vi "format_configuration_commands.vi"(8 "error in (no error)":errorcluster, 9 "True/false to 0/1?":bool, 10 "Configuration editables":T1(array[cluster])=[{"INI key name"="FieldCurrentRatio", "Configuration command"="CONF:COIL"}, {"INI key name"="HasPSwitch", "Configuration command"="CONF:PS"}, {"INI key name"="SwitchHtrCurrent", "Configuration command"="CONF:PS:CURR"}, {"INI key name"="SwitchWaitTime", "Configuration command"="CONF:PS:HTIME"}, {"INI key name"="SwitchWaitTime", "Configuration command"="CONF:PS:CTIME"}, {"INI key name"="SwitchCoolingGain", "Configuration command"="CONF:PS:CGAIN"}, {"INI key name"="StabilitySetting", "Configuration command"="CONF:STAB"}, {"INI key name"="MaxCurrent", "Configuration command"="CONF:CURR:RATING"}, {"INI key name"="MaxCurrent", "Configuration command"="CONF:CURR:LIM"}, {"INI key name"="LimitCurrent", "Configuration command"="CONF:CURR:LIM"}, {"INI key name"="QuenchDetectEnable", "Configuration command"="CONF:QU:DET"}, {"INI key name"="QuenchDetectRate", "Configuration command"="CONF:QU:RATE"}, {"INI key name"="AbsorberPresent", "Configuration command"="CONF:AB"}, {"INI key name"="SwitchPSRampRate", "Configuration command"="CONF:PS:PSRR"}], 11 "Config data in":variant) -> (0 "error out":errorcluster, 3 "Configuration commands":string[](array[string]))   [LabVIEW 2020]
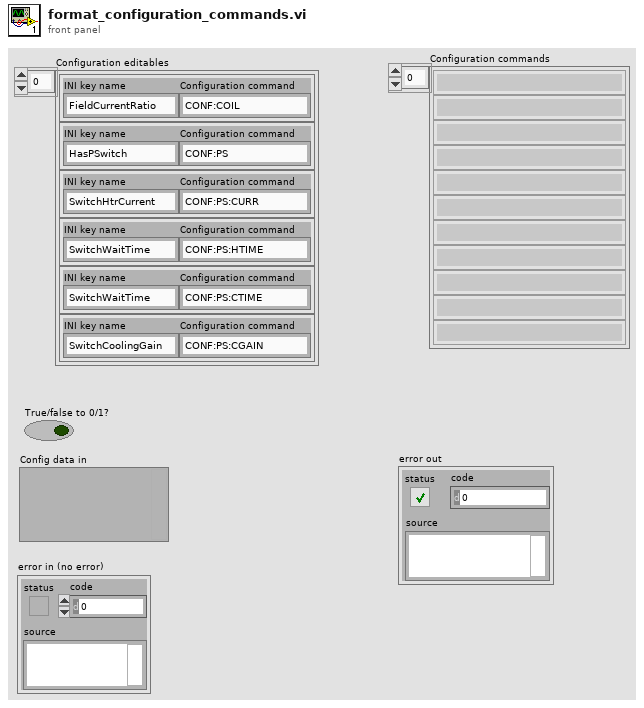
[diagram p1: front panel]
types:
  T1 = cluster{"INI key name":string, "Configuration command":string}[]
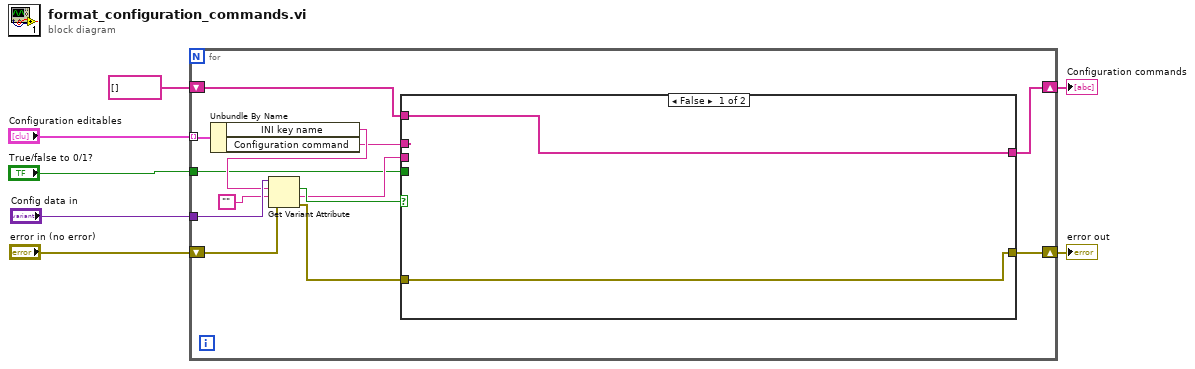
[diagram p0: block diagram]
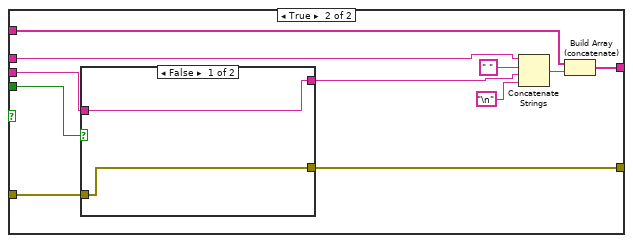
[diagram p2: hidden frame]
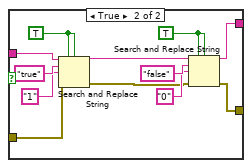
[diagram p3: hidden frame]
diagram:
  n1 = for {
    tunnel: "Configuration editables" -> [w18] mode=indexing
    tunnel: "Config data in" -> [w20]
    shift-right: [w9] -> w1
    shift-left: "error in (no error)" -> [w19]
    shift-right: [w11] -> w2
    shift-left: string[] [] ("Configuration commands") -> [w12]
    tunnel: "True/false to 0/1?" -> [w8]
    n2 = Unbundle By Name(w18) -> ("INI key name"=w17:string, "Configuration command"=w14:string)
    n3 = Get Variant Attribute(Variant=w20, name=w17, default value (empty Variant)="", error in=w19) -> (found=w15:bool, value=w13:string, error out=w10:errorcluster)  [unwired: 1 out]
    n4 = case shown="False" w15 {
      tunnel: w14 -> [_ w31]
      tunnel: w13 -> [_ w27]
      tunnel: w12 -> [w22 w29]
      tunnel: [w22 w30] -> w11
      tunnel: w10 -> [w21 w26]
      tunnel: [w21 w25] -> w9
      tunnel: w8 -> [_ w23]
      frame False {
      }
      frame True {
        n5 = case shown="False" w23 {
          tunnel: w27 -> [w35 w47]
          tunnel: w26 -> [w34 w44]
          tunnel: [w34 w37] -> w25
          tunnel: [w35 w36] -> w24
          frame False {
          }
          frame True {
            w42 = TRUE ("ignore case? (F)")
            w43 = TRUE ("ignore case? (F)")
            n6 = Search and Replace String(replace all?=w43, case sensitive?=w43, input string=w47, search string="true" ("regular expression"), replace string="1", error in=w44) -> (result string=w41:string, error out=w38:errorcluster)  [unwired: 2 in, 2 out]
            n7 = Search and Replace String(replace all?=w42, case sensitive?=w42, input string=w41, search string="false" ("regular expression"), replace string="0", error in=w38) -> (result string=w36:string, error out=w37:errorcluster)  [unwired: 2 in, 2 out]
          }
        }
        n8 = Concatenate Strings(w31, " ", w24, "\n") -> (w28:string)
        n9 = Build Array (concatenate)(w29, w28) -> (w30:string[])
      }
    }
  }
  "Configuration commands" <- w2
  "error out" <- w1
